vi "SimpleProducer.vi"(7 "Events":T1[](array[typedef]), 8 "error in (no error)":errorcluster, 9 "Partition":i32, 10 "Topic":string="qamData", 11 "Kafka Broker":string="localhost:9092") -> (0 "error out":errorcluster)   [LabVIEW 2019]
uses:
  API/KafkaConsumerEvent.ctl
  API/LVKafka.lvlib
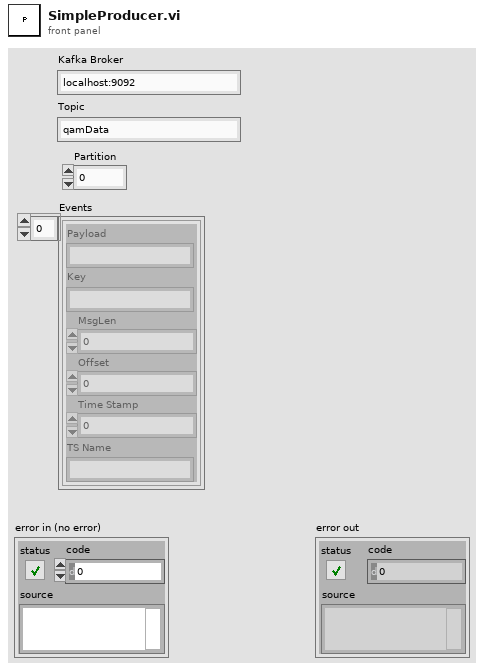
[diagram p1: front panel]
types:
  T1 = typedef "LVKafka.lvlib/KafkaConsumerEvent.ctl" = cluster{"Payload":string, "Key":string, "MsgLen":u64, "Offset":i64, "Time Stamp":i64, "TS Name":string}
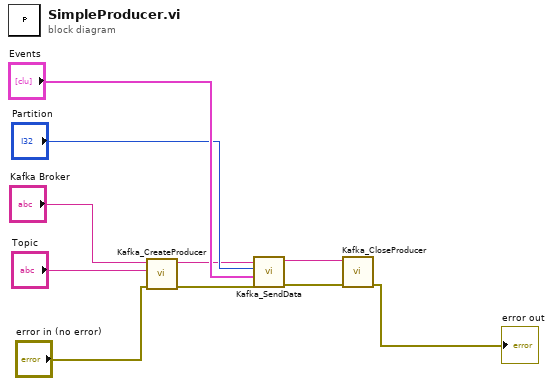
[diagram p0: block diagram]
diagram:
  n1 = call "Kafka_CreateProducer.vi"("error in (no error)"="error in (no error)", "Topic"="Topic", "Kafka Broker"="Kafka Broker") -> ("error out"=w7:errorcluster, "Producer Handle"=w4:string)  [unwired: 7 in]
  n2 = call "Kafka_SendData.vi"("error in (no error)"=w7, "Events"="Events", "Partition"="Partition", "Producer Handle"=w4) -> ("error out"=w3:errorcluster, "Producer Handle"=w2:string)  [unwired: 6 in]
  n3 = call "Kafka_CloseProducer.vi"("error in (no error)"=w3, "Producer Handle"=w2) -> ("error out"=→"error out":errorcluster)  [unwired: 8 in, 1 out]
